vi "Read Ultrasonic Sensor.vi"() -> ()   [LabVIEW 2020]
uses:
  <vilib>/High Genius/HG_WSI_Tookit/Dependencies/Library/ISQ/ISQ.lvclass
  C:/Program Files (x86)/National Instruments/LabVIEW 2020/vi.lib/High Genius/HG_WSI_Tookit/Dependencies/Library/HG_LIB/HG_LIB.lvclass
  <vilib>/High Genius/HG_WSI_Tookit/Dependencies/Library/Pulse/Pulse.lvclass
  <vilib>/Platform/TimedLoop/XDataNode/timing_clust.ctl
  <vilib>/Platform/TimedLoop/XDataNode/nitl_modes.ctl
  <vilib>/Platform/TimedLoop/XDataNode/wakeup.ctl
  <vilib>/Platform/TimedLoop/XDataNode/XDataNode.xnode
  <vilib>/Platform/TimedLoop/XDataNode/XDNodeRunTimeDep.lvlib
  <vilib>/High Genius/HG_WSI_Tookit/Dependencies/Library/HG_LIB/HG_LIB.lvclass
panel:
  out "PING right":dbl
  in  "stop":bool
  out "PING left":dbl
  # "Control Description:\nPing left: robot left ultrasonic distance sensor\nPing right: robot right ultrasonic distance sensor\n\nDescription of operation procedure steps:\n1. Running program\n2. You can hold the object in front of the ultrasonic wave and move it back and forth to observe the distance between the left and right data display of Ping"
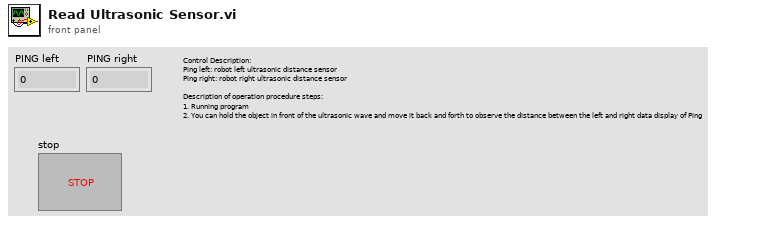
[diagram p1: front panel]
types:
  T1 = enum16{"DI", "DO", "AI", "Pulse", "PWM", "ISQ", "ENC", "CAN", "IIC", "IMU"}
  T2 = enum16{"0", "1", "2", "3", "4", "5", "6", "7", "8", "9", "10", "11", "12", "13", "14", "15", "16", "17", "18", "19", "20", "21", "22", "23", "24", "25"}
  T3 = typedef "XDNodeRunTimeDep.lvlib/timing_clust.ctl" = cluster{"Expected End [f-1]":u64, "Actual End [f-1]":u64, "Finished Late? [f-1]":bool, "Expected End [i-1]":u64, "Actual End [i-1]":u64, "Finished Late? [i-1]":bool, "Expected Start [i]":u64, "Actual Start [i]":u64, "Expected Start [f]":u64, "Actual Start [f]":u64, "Source Name":string, "Structure Name":string, "Period":i64, "Deadline":i64, "Offset":i64, "Start":i64, "Priority":i32, "Timeout":i32, "Mode":T4, "Wakeup Reason":T5, "Error":errorcluster, "Source Type":string, "Secondary Source Type":string, "Global End Time":u64, "Global Start Time":u64, "Frame Duration":u64, "Iteration Duration":u64, "Assigned CPU":i32, "I/O Scan Engine Mode":u32}
  T4 = typedef "XDNodeRunTimeDep.lvlib/nitl_modes.ctl" = enum32{"No Change", "Process missed periods, maintain original phase", "Discard missed periods, maintain original phase", "Process missed periods, ignore original phase", "Discard missed periods, ignore original phase"}
  T5 = typedef "XDNodeRunTimeDep.lvlib/wakeup.ctl" = enum32{"Normal", "Aborted", "Asynchronous wakeup", "Timing source error", "Timed loop error", "Timeout"}
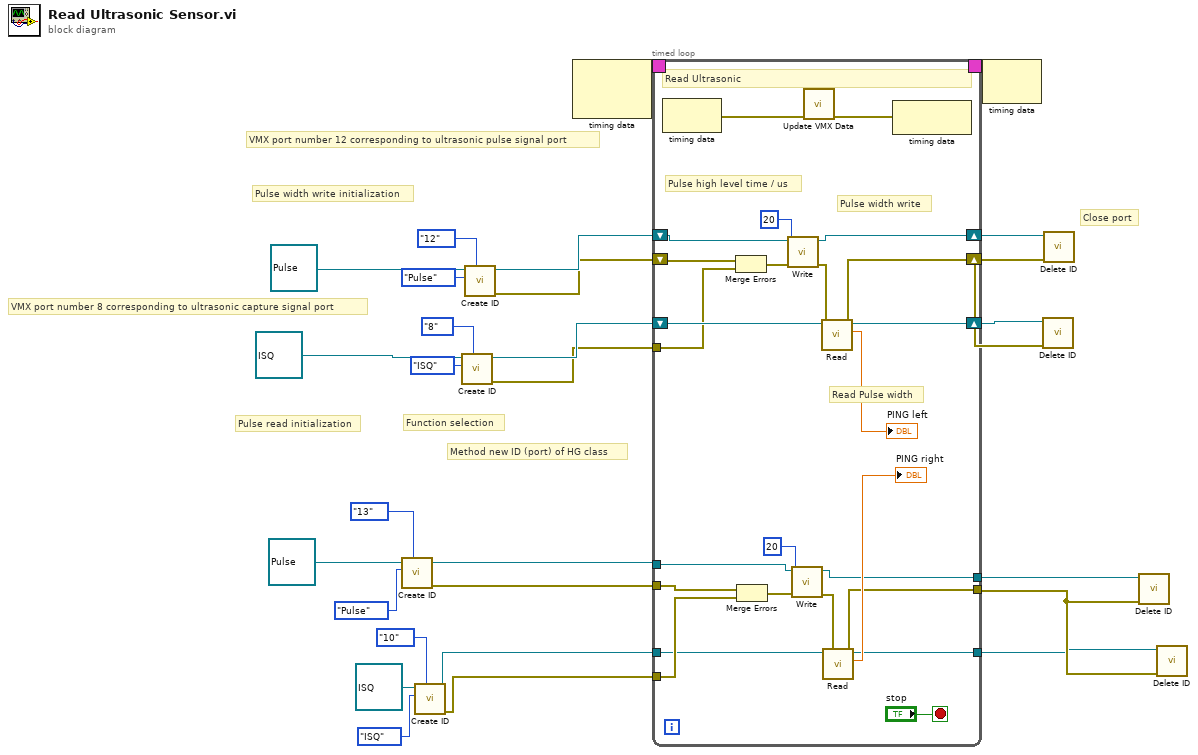
[diagram p0: block diagram]
diagram:
  # "Method new ID (port) of HG class"
  # "Function selection"
  # "Pulse read initialization"
  # "Close port"
  # "Pulse width write initialization"
  # "VMX port number 8 corresponding to ultrasonic capture signal port"
  # "VMX port number 12 corresponding to ultrasonic pulse signal port"
  n1 = call <vilib>:"Create ID.vi"("NO"=T2."13", "Function"=T1."Pulse", "HG_LIB in"=refnum<class "Pulse.lvclass"> refnum ("VMX Library.lvlib:Pulse.lvclass")) -> ("error out"=w21:errorcluster, "HG_LIB out"=w26:refnum<class "Pulse.lvclass">)  [unwired: 7 in]
  n2 = call <vilib>:"Create ID.vi"("NO"=T2."10", "Function"=T1."ISQ", "HG_LIB in"=refnum<class "ISQ.lvclass"> refnum ("ISQ.lvclass")) -> ("error out"=w22:errorcluster, "HG_LIB out"=w23:refnum<class "ISQ.lvclass">)  [unwired: 7 in]
  n3 = call <vilib>:"Create ID.vi"("NO"=T2."8", "Function"=T1."ISQ", "HG_LIB in"=refnum<class "ISQ.lvclass"> refnum ("ISQ.lvclass")) -> ("error out"=w4:errorcluster, "HG_LIB out"=w13:refnum<class "ISQ.lvclass">)  [unwired: 7 in]
  n4 = call <vilib>:"Create ID.vi"("NO"=T2."12", "Function"=T1."Pulse", "HG_LIB in"=refnum<class "Pulse.lvclass"> refnum ("VMX Library.lvlib:Pulse.lvclass")) -> ("error out"=w11:errorcluster, "HG_LIB out"=w15:refnum<class "Pulse.lvclass">)  [unwired: 7 in]
  n5 = node-c288() -> (w28:T3)  [unwired: 2 in]
  n6 = timed-loop {
    shift-right: [w35] -> w10
    shift-left: w15 -> [w36]
    shift-right: [w52] -> w12
    shift-left: w13 -> [w53]
    shift-right: [w51] -> w9
    shift-left: w11 -> [w48]
    timing: w28 -> [_]
    timing-out: [_] -> w27
    tunnel: w4 -> [w47]
    tunnel: w21 -> [w43]
    tunnel: w22 -> [w42]
    tunnel: w23 -> [w41]
    tunnel: [w40] -> w24
    tunnel: [w39] -> w25
    tunnel: w26 -> [w33]
    tunnel: [w32] -> w1
    stop <- "stop" stop-if-true
    # "Read Pulse width"
    # "Pulse width write"
    # "Pulse high level time / us"
    # "Read Ultrasonic"
    n7 = node-c288() -> (w46:errorcluster)  [unwired: 1 in]
    n8 = Merge Errors(w48, w47) -> (w38:errorcluster)
    n9 = Merge Errors(w43, w42) -> (w31:errorcluster)
    n10 = call <vilib>:"Write.vi"("error in (no error)"=w38, "Pulse"=20 ("Pluse"), "Pulse in"=w36) -> ("error out"=w34:errorcluster, "Pulse out"=w35:refnum<class "Pulse.lvclass">)  [unwired: 7 in]
    n11 = call <vilib>:"Write.vi"("error in (no error)"=w31, "Pulse"=20 ("Pluse"), "Pulse in"=w33) -> ("error out"=w29:errorcluster, "Pulse out"=w32:refnum<class "Pulse.lvclass">)  [unwired: 7 in]
    n12 = call <vilib>:"Update VMX Data.vi"("error in (no error)"=w46) -> ("error out"=w45:errorcluster)  [unwired: 10 in]
    n13 = call <vilib>:"Read.vi"("error in (no error)"=w34, "ISQ in"=w53) -> ("error out"=w51:errorcluster, "PING"=→"PING left":dbl, "ISQ out"=w52:refnum<class "ISQ.lvclass">)  [unwired: 7 in]
    n14 = call <vilib>:"Read.vi"("error in (no error)"=w29, "ISQ in"=w41) -> ("error out"=w39:errorcluster, "PING"=→"PING right":dbl, "ISQ out"=w40:refnum<class "ISQ.lvclass">)  [unwired: 7 in]
    n15 = node-c288(w45) -> ()  [unwired: 1 out]
  }
  n16 = node-c288(w27) -> ()  [unwired: 1 out]
  n17 = call <vilib>:"Delete ID.vi"("error in (no error)"=w9, "HG_LIB in"=w12) -> ()  [unwired: 8 in, 2 out]
  n18 = call <vilib>:"Delete ID.vi"("error in (no error)"=w9, "HG_LIB in"=w10) -> ()  [unwired: 8 in, 2 out]
  n19 = call <vilib>:"Delete ID.vi"("error in (no error)"=w25, "HG_LIB in"=w1) -> ()  [unwired: 8 in, 2 out]
  n20 = call <vilib>:"Delete ID.vi"("error in (no error)"=w25, "HG_LIB in"=w24) -> ()  [unwired: 8 in, 2 out]
